vi "generate reference signal.vi"(8 "error in (no error)":errorcluster, 11 "mass-spring-damper in":refnum<class "mass-spring-damper.lvclass">) -> (0 "error out":errorcluster, 2 "Reference Array":cluster{"Time":dbl[], "Reference":dbl[]}, 3 "mass-spring-damper out":refnum<class "mass-spring-damper.lvclass">)   [LabVIEW 2025, in "mass-spring-damper.lvclass"]
uses:
  mass-spring-damper.lvclass
  mass-spring-damper.lvclass/mass-spring-damper.ctl
panel:
  out "Time":dbl[](array[numeric])
  out "Reference":dbl[](array[numeric])
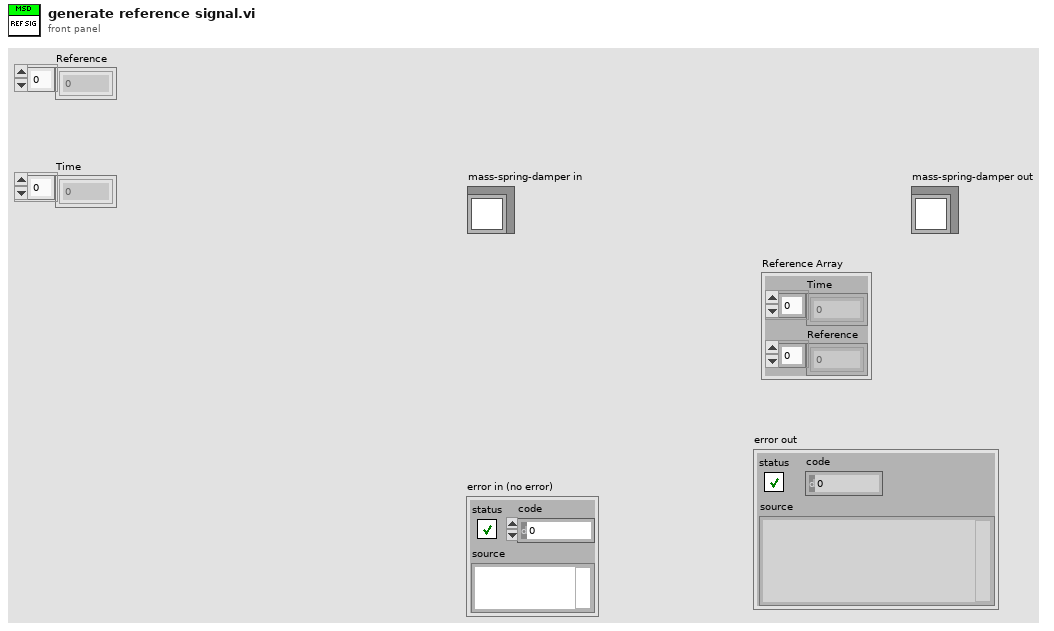
[diagram p1: front panel]
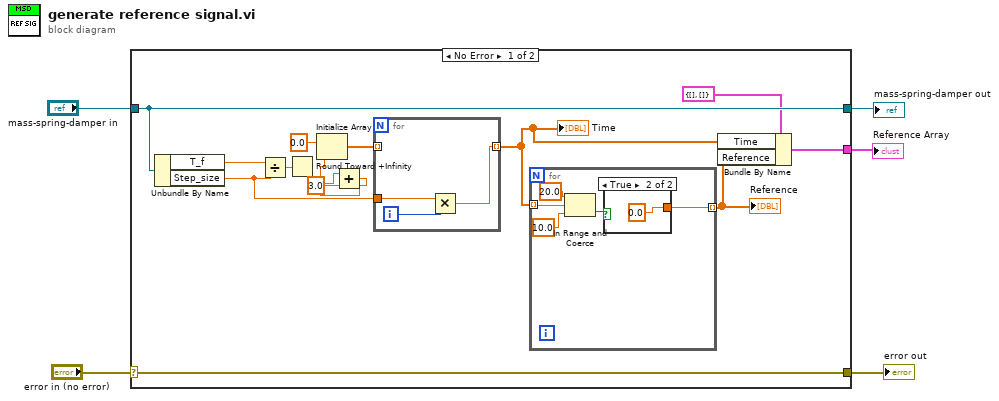
[diagram p0: block diagram]
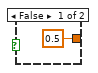
[diagram p2: hidden frame]
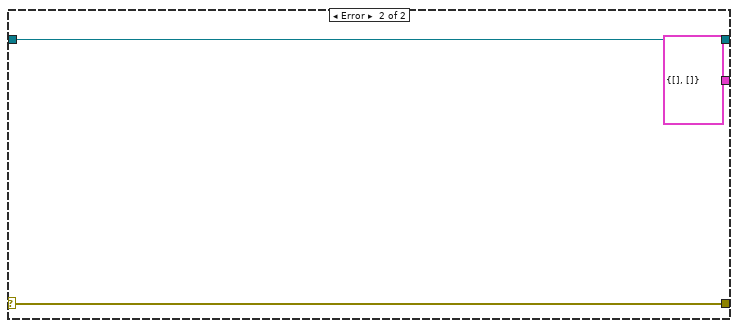
[diagram p3: hidden frame]
diagram:
  n1 = case shown="No Error" "error in (no error)" {
    selector: "error in (no error)" -> [w19 w32]
    tunnel: [w19 w32] -> w3
    tunnel: [w18 w31] -> w1
    tunnel: "mass-spring-damper in" -> [w18 w31]
    tunnel: [w10 cluster{"Time":dbl[], "Reference":dbl[]} {"Time"=[], "Reference"=[]} ("cluster")] -> w2
    frame No Error {
      n2 = Unbundle By Name(w18) -> ("T_f"=w17:dbl, "Step_size"=w14:dbl)
      n3 = Divide(x=w17, y=w14) -> (x/y=w9:dbl)
      n4 = Round Toward +Infinity(x=w9) -> (ceil(x): smallest int >= x=w8:dbl)
      n5 = Add(x=w8, y=3.0) -> (x+y=w7:dbl)
      n6 = Initialize Array(0.0 ("element"), w7) -> (w15:dbl[])
      n7 = for {
        tunnel: w15 -> [_] mode=indexing
        tunnel: w14 -> [w28]
        tunnel: [w27] -> w12 mode=indexing
        i -> [w29]
        n8 = Multiply(x=w28, y=w29) -> (x*y=w27:dbl)
      }
      "Time" <- w12
      n9 = for {
        tunnel: w12 -> [w24] mode=indexing
        tunnel: [w20] -> w11 mode=indexing
        n10 = In Range and Coerce(upper limit=20.0, x=w24, lower limit=10.0) -> (In Range?=w21:bool)  [unwired: 1 out]
        n11 = case shown="True" w21 {
          tunnel: [0.5 0.0] -> w20
          frame False {
          }
          frame True {
          }
        }
      }
      "Reference" <- w11
      n12 = Bundle By Name(cluster=cluster{"Time":dbl[], "Reference":dbl[]} {"Time"=[], "Reference"=[]}, "Time"=w12, "Reference"=w11) -> (w10:cluster{"Time":dbl[], "Reference":dbl[]})
    }
    frame Error {
    }
  }
  "error out" <- w3
  "mass-spring-damper out" <- w1
  "Reference Array" <- w2
